vi "Build Connection Strings.vi"(0 "Vector Paths in":refnum<class "Vector Abstract Path.lvclass">[](array[class]), 5 "Start Index":i32, 7 "Subgroup Size":i32, 11 "error in (no error)":errorcluster) -> (4 "Vector Paths out":refnum<class "Vector Abstract Path.lvclass">[](array[class]), 6 "Connection Strings":string[](array[string]), 15 "error out":errorcluster)   [LabVIEW 2023, in "RFFixtureCharact.Public.lvlib" / "Vector Abstract Path.lvclass"]
uses:
  Vector Abstract Path.lvclass
  C:/rfcal/AuxTools/STSRFFixtureCharactUtility/Source/Code Modules/Common/Base Classes/Path/Path.lvclass
  Vector Abstract Path.lvclass/Vector Abstract Path.ctl
  Properties/Read Cal Standard Port.vi
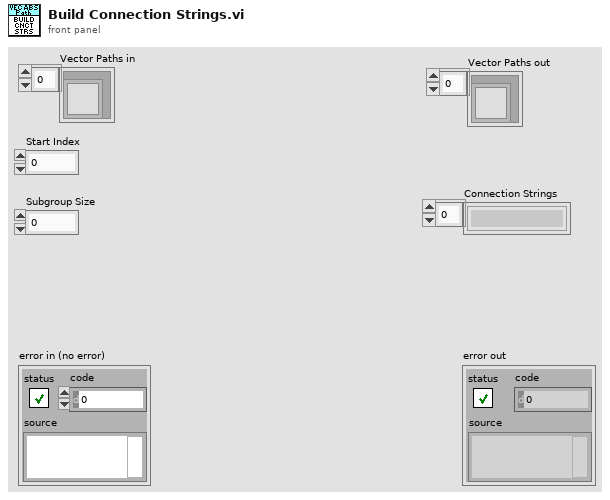
[diagram p1: front panel]
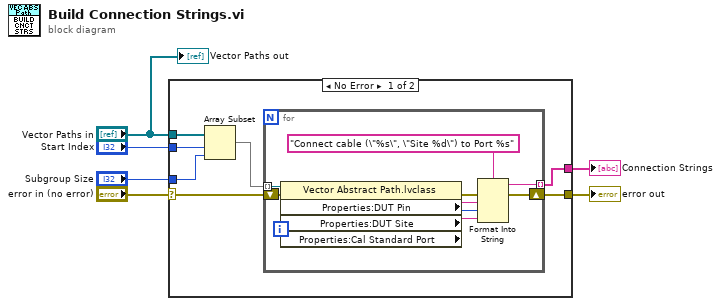
[diagram p0: block diagram]
diagram:
  n1 = case shown="No Error" "error in (no error)" {
    selector: "error in (no error)" -> [w13 w23]
    tunnel: [w12 w23] -> w5
    tunnel: "Vector Paths in" -> [w10 _]
    tunnel: [w11 _] -> w4
    tunnel: "Subgroup Size" -> [w8 _]
    tunnel: "Start Index" -> [w7 _]
    frame No Error {
      n2 = Array Subset(array=w10, index=w7, length=w8) -> (w9:refnum<class "Vector Abstract Path.lvclass">[])
      n3 = for {
        shift-right: [w20] -> w12
        shift-left: w13 -> [w17]
        tunnel: w9 -> [w18] mode=indexing
        tunnel: [w19] -> w11 mode=indexing
        n4 = property class="Vector Abstract Path.lvclass"(reference=w18, error in=w17) -> (error out=w22:errorcluster, "Properties:DUT Pin"=w16:string, "Properties:DUT Site"=w15:i32, "Properties:Cal Standard Port"=w14:string)  [unwired: 1 out]
        n5 = Format Into String(format string="Connect cable (\"%s\", \"Site %d\") to Port %s", error in=w22, w16, w15, w14) -> (resulting string=w19:string, error out=w20:errorcluster)  [unwired: 1 in]
      }
    }
    frame Error {
    }
  }
  "error out" <- w5
  "Connection Strings" <- w4
  "Vector Paths out" <- "Vector Paths in"
